vi "parse_gulton_number.vi"(0 "Stripped Gulton String":string) -> (1 "value":dbl format="%.2f", 4 "Error notes":string)   [LabVIEW 2010]
panel:
  out "Range":i32
  out "Quantity":i32
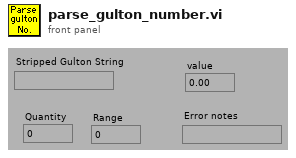
[diagram p1: front panel]
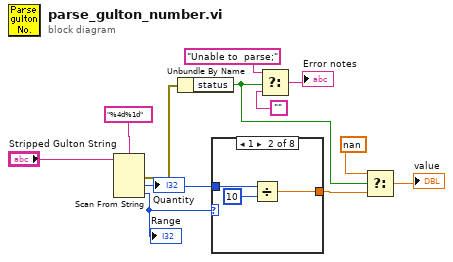
[diagram p0: block diagram]
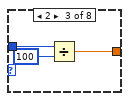
[diagram p3: hidden frame]
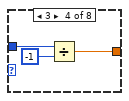
[diagram p4: hidden frame]
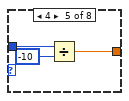
[diagram p5: hidden frame]
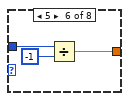
[diagram p6: hidden frame]
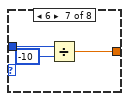
[diagram p7: hidden frame]
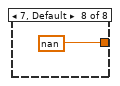
[diagram p8: hidden frame]
diagram:
  n1 = Scan From String(format string="%4d%1d", input string="Stripped Gulton String") -> (error out=w5:errorcluster, output 1=w9:i32, output 2=w10:i32)  [unwired: 4 in, 2 out]
  "Quantity" <- w9
  "Range" <- w10
  n2 = Unbundle By Name(w5) -> ("status"=w4:bool)
  n3 = case shown="1" w10 {
    tunnel: w9 -> [w13 w16 w19 w22 w25 w28 w31 _]
    tunnel: [w13 w14 w17 w20 w23 w26 w29 nan] -> w3
    frame 0 {
    }
    frame 1 {
      n4 = Divide(x=w16, y=10) -> (x/y=w14:dbl)
    }
    frame 2 {
      n5 = Divide(x=w19, y=100) -> (x/y=w17:dbl)
    }
    frame 3 {
      n6 = Divide(x=w22, y=-1) -> (x/y=w20:dbl)
    }
    frame 4 {
      n7 = Divide(x=w25, y=-10) -> (x/y=w23:dbl)
    }
    frame 5 {
      n8 = Divide(x=w28, y=-1) -> (x/y=w26:dbl)
    }
    frame 6 {
      n9 = Divide(x=w31, y=-10) -> (x/y=w29:dbl)
    }
    frame 7, Default {
    }
  }
  n10 = Select(t="Unable to  parse;", s=w4, f="") -> (s? t:f=→"Error notes":string)
  n11 = Select(t=nan, s=w4, f=w3) -> (s? t:f=→"value":dbl)
